vi "Save TS DAC Results.vi"(8 "error in":errorcluster, 11 "LNG Boiling Test Stand in":refnum<class "LNG Boiling Test Stand.lvclass">) -> (0 "error out":errorcluster, 3 "LNG Boiling Test Stand out":refnum<class "LNG Boiling Test Stand.lvclass">)   [LabVIEW 2019, in "Test Stands.lvlib" / "LNG Boiling Test Stand.lvclass"]
uses:
  LNG Boiling Test Stand.lvclass
  C:/Users/krio/Documents/LV_Projects/TestStand/App/Generic Test Stand/Generic Test Stand.lvclass
  Results/LNG Boiling Results/LNG Boiling Results.lvclass
  Results/Results Method.ctl
  Generic Test Stand/Generic Test Stand.lvclass/Generic Test Stand.ctl
  DAC/DAC.lvclass
  Results/Results.lvlib
  Generic Test Stand/Generic Test Stand.lvclass
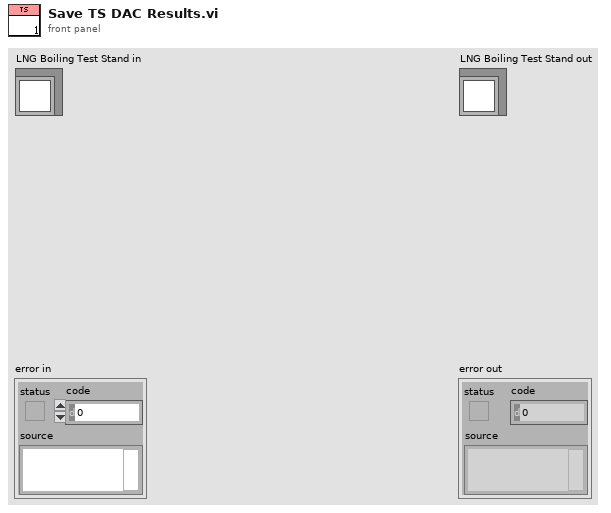
[diagram p1: front panel]
types:
  T1 = typedef "Results.lvlib/Results Method.ctl" = enum16{"Get", "Set"}
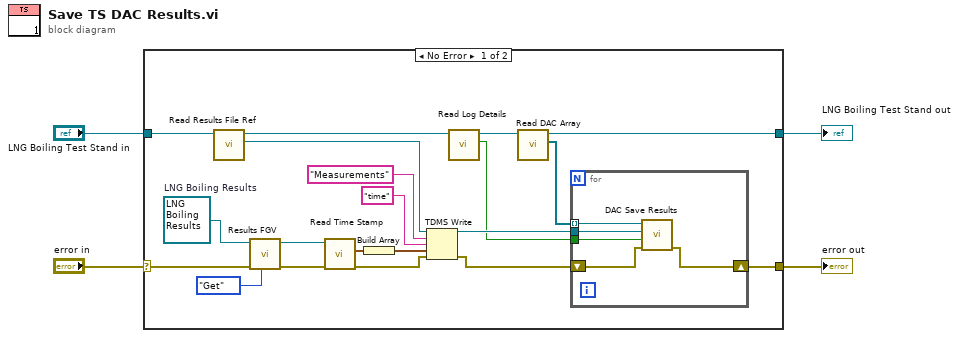
[diagram p0: block diagram]
diagram:
  n1 = case shown="No Error" "error in" {
    selector: "error in" -> [w15 w31]
    tunnel: "LNG Boiling Test Stand in" -> [w22 w30]
    tunnel: [w11 w30] -> w2
    tunnel: [w8 w31] -> w1
    frame No Error {
      w24 = refnum<class "LNG Boiling Results.lvclass"> refnum  # LNG Boiling Results
      n2 = call "Read Results File Ref.vi"("Generic Test Stand in"=w22) -> ("Results File Ref"=w20:refnum<k34>, "Generic Test Stand out"=w7:refnum<class "LNG Boiling Test Stand.lvclass">)  [unwired: 8 in, 1 out]
      n3 = call-dynamic "Results FGV.vi"("Method"=Results_Method."Get", "error in"=w15, "LNG Boiling Results in"=w24) -> ("error out"=w14:errorcluster, "LNG Boiling Results out"=w21:refnum<class "LNG Boiling Results.lvclass">)  [unwired: 7 in]
      n4 = call-dynamic "Read Time Stamp.vi"("error in (no error)"=w14, "Results in"=w21) -> ("error out"=w13:errorcluster, "Time Stamp"=w19:timestamp)  [unwired: 7 in, 1 out]
      n5 = Build Array(w19) -> (w18:timestamp[])
      n6 = TDMS Write(0:w20, 5:"Measurements" ("group name in (Untitled)"), 7:"time" ("group name in (Untitled)"), 9:w18, 11:w13) -> (4:w12:refnum<k34>, 15:w9:errorcluster)  [unwired: 1 in, 2 out]
      n7 = call "Read Log Details.vi"("Generic Test Stand in"=w7) -> ("Log Details"=w5:bool, "Generic Test Stand out"=w6:refnum<class "LNG Boiling Test Stand.lvclass">)  [unwired: 8 in, 1 out]
      n8 = call "Read DAC Array.vi"("Generic Test Stand in"=w6) -> ("DAC Array"=w10:refnum<class "DAC.lvclass">[], "Generic Test Stand out"=w11:refnum<class "LNG Boiling Test Stand.lvclass">)  [unwired: 8 in, 1 out]
      n9 = for {
        tunnel: w10 -> [w29] mode=indexing
        shift-right: [w26] -> w8
        shift-left: w9 -> [w27]
        tunnel: w12 -> [w28]
        tunnel: w5 -> [w25]
        n10 = call-dynamic "DAC Save Results.vi"("error in"=w27, "Log Details?"=w25, "tdms file"=w28, "DAC in"=w29) -> ("error out"=w26:errorcluster)  [unwired: 7 in]
      }
    }
    frame Error {
    }
  }
  "error out" <- w1
  "LNG Boiling Test Stand out" <- w2
